vi "PVCAM_GetLastError.vi"() -> (3 "return type 2":string)   [LabVIEW 2021]
uses:
  Windows/System32/pvcam64.dll
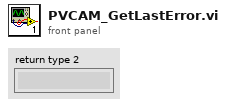
[diagram p1: front panel]
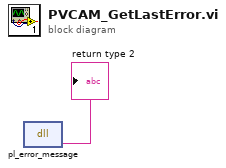
[diagram p0: block diagram]
diagram:
  n1 = dll-call lib="C:/Windows/System32/pvcam64.dll" fn="pl_error_message"() -> ("return type"=→"return type 2":string)  [unwired: 3 in, 2 out]
